vi "Select Object.vi"(10 "Coords":T1, 11 "Scene in":refnum<class "Scene.lvclass">) -> (3 "Active Object":i32)   [LabVIEW 2020, in "Scene.lvclass"]
uses:
  Scene.lvclass
  Scene.lvclass/Scene.ctl
  Graphics/Libraries/3D/Vector 3D.ctl
  Graphics/Libraries/3D/3D.lvlib
  <vilib>/Analysis/NI_AAL_Geometry.lvlib
  <vilib>/Analysis/geometry.llb/Point in Polygon (Scalar).vi
  <userlib>/_OpenG.lib/array/array.llb/openg_array.lvlib
  <userlib>/_OpenG.lib/array/array.llb/Sort 1D Array (SGL)__ogtk.vi
  <vilib>/Utility/miscctls.llb/LVPoint32TypeDef.ctl
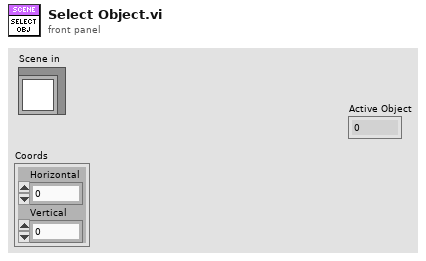
[diagram p1: front panel]
types:
  T1 = typedef "LVPoint32TypeDef.ctl" = cluster{"Horizontal":i32, "Vertical":i32}
  T2 = typedef "3D.lvlib/Vector 3D.ctl" = cluster{"x":sgl, "y":sgl, "z":sgl}
  T3 = typedef "Raster.lvlib/Rectangle Dimensions.ctl" = cluster{"Width":u32, "Height":u32}
  T4 = typedef "3D.lvlib/Object.ctl" = cluster{"Triangles":T5[], "Transform":T10, "Name":string, "Alpha Blending Enabled":bool, "Alpha":dbl, "Turntable Enabled":bool, "Material":T8}
  T5 = typedef "3D.lvlib/Triangle.ctl" = cluster{"Vertex 1":T6, "Vertex 2":T6, "Vertex 3":T6, "Alpha":dbl, "Alpha Blending Enabled":bool, "Colour":u32, "Material":T8}
  T6 = typedef "3D.lvlib/Vertex.ctl" = cluster{"Position":T2, "UV":T7, "Colour":u32}
  T7 = typedef "Raster.lvlib/UV.ctl" = cluster{"u":sgl, "v":sgl}
  T8 = typedef "3D.lvlib/Material.ctl" = cluster{"Diffuse Colour":u32, "Texture":T9}
  T9 = typedef "Raster.lvlib/Texture.ctl" = cluster{"Pixels":refnum<data-value>, "Size":T3}
  T10 = typedef "3D.lvlib/Transform.ctl" = cluster{"Position":T2, "Rotation":T2, "Scale":T2}
  T11 = typedef "NI_AAL_Geometry.lvlib/Point in Polygon Position.ctl" = u16
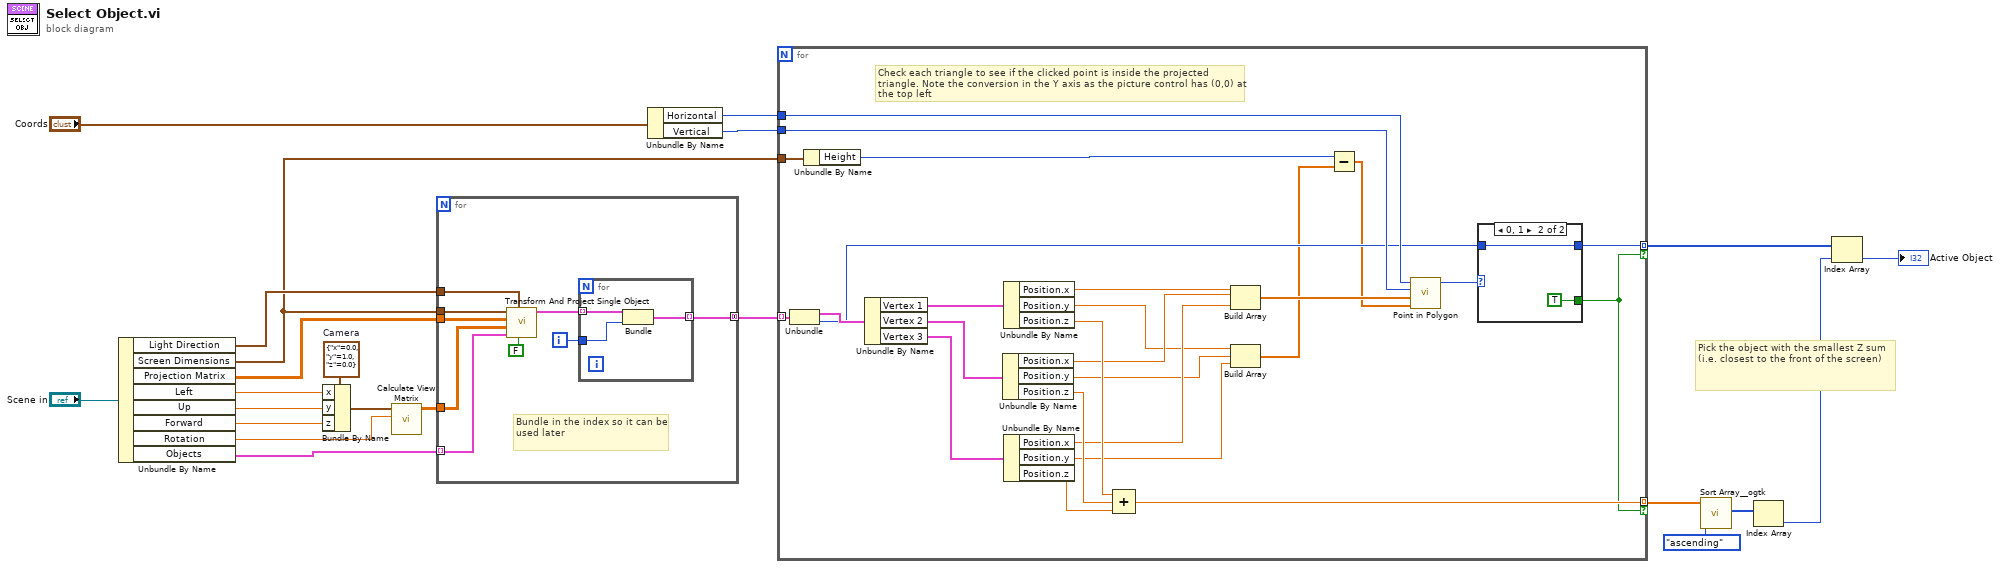
[diagram p0: block diagram]
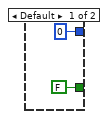
[diagram p2: hidden frame]
diagram:
  w22 = T2 {"x"=0.0, "y"=1.0, "z"=0.0}  # Camera
  # "Pick the object with the smallest Z sum (i.e. closest to the front of the screen)"
  n1 = Unbundle By Name("Scene in") -> ("Light Direction"=w13:T2, "Screen Dimensions"=w8:T3, "Projection Matrix"=w14:sgl[][], "Left"=w17:sgl, "Up"=w18:sgl, "Forward"=w21:sgl, "Rotation"=w19:sgl, "Objects"=w15:T4[])
  n2 = Bundle By Name(cluster=w22, "x"=w17, "y"=w18, "z"=w21) -> (w16:T2)
  n3 = call "Calculate View Matrix.vi"("Camera Rotation"=w19, "Camera Position"=w16) -> ("View Matrix"=w20:sgl[][])  [unwired: 9 in]
  n4 = for {
    tunnel: w20 -> [w29]
    tunnel: w15 -> [w24] mode=indexing
    tunnel: w8 -> [w31]
    tunnel: w14 -> [w30]
    tunnel: w13 -> [w28]
    tunnel: [w25] -> w12 mode=concatenating
    i -> [w26]
    # "Bundle in the index so it can be used later"
    n5 = call "Transform And Project Single Object.vi"("Backface Culling Enabled"=FALSE, "Light Direction"=w28, "Object"=w24, "View Matrix"=w29, "Projection Matrix"=w30, "Screen Dimensions"=w31) -> ("Triangles"=w27:T5[])  [unwired: 5 in]
    n6 = for {
      tunnel: w27 -> [w34] mode=indexing
      tunnel: w26 -> [w33]
      tunnel: [w32] -> w25 mode=indexing
      n7 = Bundle("Cluster"=w34, w33) -> (w32:cluster{"Cluster":T5, i32})  [unwired: 1 in]
    }
  }
  n8 = Unbundle By Name("Coords") -> ("Horizontal"=w10:i32, "Vertical"=w9:i32)
  n9 = for {
    tunnel: w12 -> [w56] mode=indexing
    tunnel: [w57] -> w7 mode=indexing if=w35
    tunnel: w10 -> [w47]
    tunnel: w9 -> [w46]
    tunnel: [w44] -> w4 mode=indexing if=w35
    tunnel: w8 -> [w42]
    # "Check each triangle to see if the clicked point is inside the projected triangle. Note the conversion in the Y axis as the picture control has (0,0) at the top left"
    n10 = Unbundle(w56) -> ("Cluster"=w55:T5, w43:i32)
    n11 = Unbundle By Name(w42) -> ("Height"=w41:u32)
    n12 = Unbundle By Name(w55) -> ("Vertex 1"=w38:T6, "Vertex 2"=w37:T6, "Vertex 3"=w36:T6)
    n13 = Unbundle By Name(w37) -> ("Position.x"=w53:sgl, "Position.y"=w49:sgl, "Position.z"=w59:sgl)
    n14 = Unbundle By Name(w38) -> ("Position.x"=w54:sgl, "Position.y"=w50:sgl, "Position.z"=w60:sgl)
    n15 = Unbundle By Name(w36) -> ("Position.x"=w52:sgl, "Position.y"=w48:sgl, "Position.z"=w58:sgl)
    n16 = Compound Arithmetic op=ADD(w60, w59, w58) -> (w57:sgl)
    n17 = Build Array(w54, w53, w52) -> (w51:sgl[])
    n18 = Build Array(w50, w49, w48) -> (w40:sgl[])
    n19 = Subtract(x=w41, y=w40) -> (x-y=w39:sgl[])
    n20 = call-poly <vilib>:"Point in Polygon.vi"("Polygon Y"=w39, "Polygon X"=w51, "y"=w46, "x"=w47) -> ("position"=w45:T11)  [unwired: 6 in, 1 out]
    n21 = case shown="0, 1" w45 {
      tunnel: [0 w64] -> w44
      tunnel: w43 -> [_ w64]
      tunnel: [FALSE TRUE] -> w35
      frame Default {
      }
      frame 0, 1 {
      }
    }
  }
  n22 = call-poly <userlib>:"Sort Array__ogtk.vi"("Order"=enum16{"ascending", "descending"}."ascending", "Array in"=w7) -> ("Sorted Pointers"=w5:i32[])  [unwired: 8 in, 1 out]
  n23 = Index Array(array=w5) -> (element=w3:i32)  [unwired: 1 in]
  n24 = Index Array(array=w4, index=w3) -> (element=→"Active Object":i32)
